vi "Register.vi"(11 "Base Event in":refnum<class "Base Event.lvclass">) -> (2 "Registration":refnum<event-registration>, 3 "Base Event out":refnum<class "Base Event.lvclass">)   [LabVIEW 2021, in "jettl.lvlib" / "Base Event.lvlib" / "Base Event.lvclass"]
uses:
  Base Event.lvclass
  Msg Type Strategy/Event Msg Type Strategy/Event Msg Type Strategy.lvclass
  Addresses/Addresses.lvlib
  Msg Strategy/Msg Strategy.lvclass
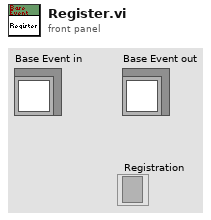
[diagram p1: front panel]
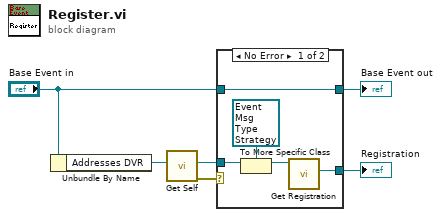
[diagram p0: block diagram]
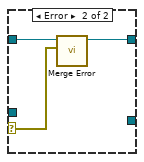
[diagram p2: hidden frame]
diagram:
  n1 = Unbundle By Name("Base Event in") -> ("Addresses DVR"=w5:refnum<data-value>)
  n2 = call "Get Self.vi"("Addresses DVR"=w5) -> ("error out"=w3:errorcluster, "Self"=w4:refnum<class "Msg Type Strategy.lvclass">)  [unwired: 9 in]
  n3 = case shown="No Error" w3 {
    selector: w3 -> [_ w12]
    tunnel: [w11 _] -> w6
    tunnel: w4 -> [w10 _]
    tunnel: [w7 w13] -> w2
    tunnel: "Base Event in" -> [w7 w14]
    frame No Error {
      n4 = To More Specific Class(target class=refnum<class "Event Msg Type Strategy.lvclass"> refnum ("jettl.lvlib:Msg Type Strategy.lvlib:Event Msg Type Strategy.lvclass"), reference=w10) -> (specific class reference=w9:refnum<class "Event Msg Type Strategy.lvclass">)  [unwired: 1 in, 1 out]
      n5 = call "Get Registration.vi"("Event Msg Type Strategy in"=w9) -> ("Registration"=w11:refnum<event-registration>)  [unwired: 10 in]
    }
    frame Error {
      n6 = call-dynamic "Merge Error.vi"("Error"=w12, "Base Event in"=w14) -> ("Base Event out"=w13:refnum<class "Base Event.lvclass">)  [unwired: 9 in]
    }
  }
  "Registration" <- w6
  "Base Event out" <- w2
